vi "Send_SCP.vi"(8 "error in (no error)":errorcluster, 10 "SCP_Cluster_In":T1, 11 "TCP Network Connection in":refnum<k5>) -> (0 "error out":errorcluster, 1 "CMD Msg":string, 2 "SCP_Cluster_Out":T1, 3 "TCP Network Connection out":refnum<k5>)   [LabVIEW 2018, in "SCP.lvlib"]
uses:
  SCP.lvlib
  Engine/Type/SCP_Cluster.ctl
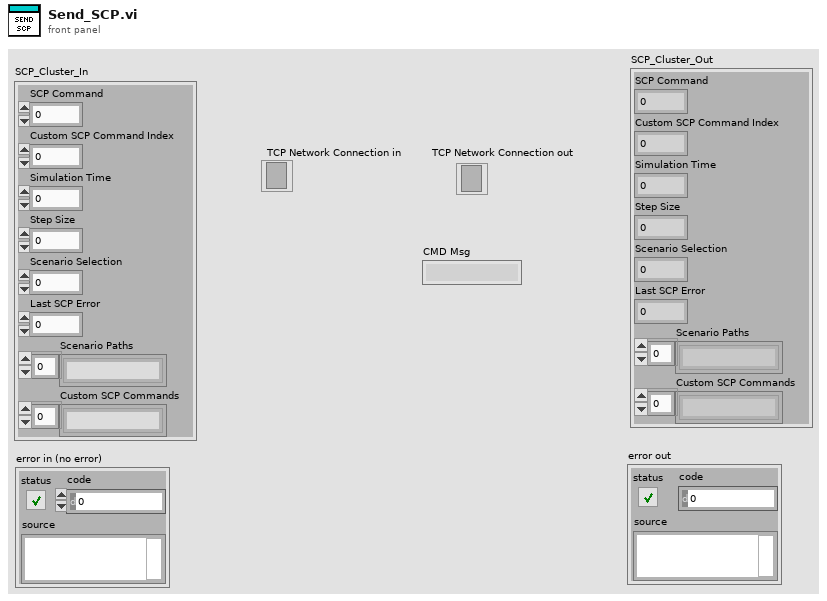
[diagram p1: front panel]
types:
  T1 = typedef "SCP.lvlib/SCP_Cluster.ctl" = cluster{"SCP Command ":i32, "Custom SCP Command Index":i32, "Simulation Time":i32, "Step Size":i32, "Scenario Selection":i32, "Last SCP Error":i32, "Scenario Paths":string[], "Custom SCP Commands":string[]}
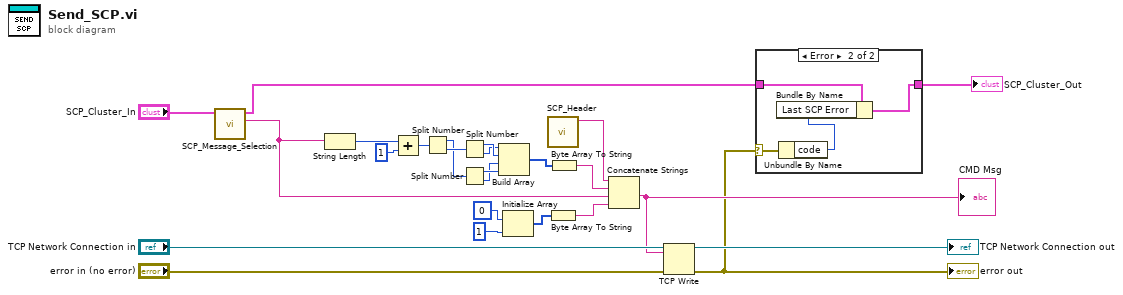
[diagram p0: block diagram]
diagram:
  n1 = call "SCP_Message_Selection.vi"("SCP_Cluster_In"="SCP_Cluster_In") -> ("SCP_Command_String_Out"=w4:string, "SCP_Cluster_Out"=w3:T1)  [unwired: 9 in]
  n2 = String Length(string=w4) -> (length=w16:i32)
  n3 = Add(x=w16, y=1) -> (x+y=w20:i32)
  n4 = Split Number(x=w20) -> (hi(x)=w6:u16, lo(x)=w7:u16)
  n5 = Split Number(x=w7) -> (hi(x)=w13:u8, lo(x)=w12:u8)
  n6 = Split Number(x=w6) -> (hi(x)=w15:u8, lo(x)=w14:u8)
  n7 = Build Array(w12, w13, w14, w15) -> (w1:u8[])
  n8 = Initialize Array(u8 0, 1 ("dimension size")) -> (w10:u8[])
  n9 = call "SCP_Header.vi"() -> ("Header Output"=w19:string)  [unwired: 11 in]
  n10 = Byte Array To String(unsigned byte array=w10) -> (string=w18:string)
  n11 = Byte Array To String(unsigned byte array=w1) -> (string=w8:string)
  n12 = Concatenate Strings(w19, w8, w4, w18) -> (w21:string)
  "CMD Msg" <- w21
  n13 = TCP Write(connection ID="TCP Network Connection in", data in=w21, error in (no error)="error in (no error)") -> (connection ID out=→"TCP Network Connection out":refnum<k5>, error out=w5:errorcluster)  [unwired: 1 in, 1 out]
  "error out" <- w5
  n14 = case shown="Error" w5 {
    selector: w5 -> [_ w30]
    tunnel: w3 -> [w26 w28]
    tunnel: [w26 w27] -> w2
    frame No Error {
    }
    frame Error {
      n15 = Unbundle By Name(w30) -> ("code"=w29:i32)
      n16 = Bundle By Name(cluster=w28, "Last SCP Error"=w29) -> (w27:T1)
    }
  }
  "SCP_Cluster_Out" <- w2
